vi "Help communication.vi"() -> ()   [LabVIEW 2018]
panel:
  out "EN help":string="The Channel selector is used to choose the type of communication between S4ICS and its clients.\nThe \"Inner TCP/IP\" option is implemented within the S4ICS program while the others are in the \"S4ICS InterComm.vi\" VI, opened and closed by S4ICS transparently for the user, unless the Local Panel option is selected. Local Panel is a GUI that allows local interactivity with SPARC4, replacing remote clients.\nThe Address, Port and Timeout configuration parameters are shared with TCP/IP, MQTT and ZeroMQ protocols.\nMQTT\nMQTT clients must connect to the broker indicated in Address and publish to topic \"lna/instrument/sparc4/command\" to send commands and subscribe to topic \"lna/instrument/sparc4/status\" to receive status message from S4ICS.\nZeroMQ\nZeroMQ customers..." caption="COMMUNICATION SELECTOR"
  out "PT help":string="O seletor Channel é usado para escolher o tipo de comunicação entre o S4ICS e seus clientes.\nA opção \"Inner TCP/IP\" está implementada dentro do programa S4ICS enquanto as demais no VI \"S4ICS InterComm.vi\", aberto e fechado pelo S4ICS de forma transparente para o usuário, exceto se a opção Local Panel for selecionada. Local Panel é uma GUI que permite interatividade local com o SPARC4, substituindo clientes remotos.\nOs parâmetros de configuração Address, Port e Timeout são compartilhados com os protocolos TCP/IP, MQTT e ZeroMQ.\nMQTT\nOs clientes MQTT devem se conectar ao broker indicado em Address e publicar no tópico \"lna/instrument/sparc4/command\" para enviar comandos e assinar o tópico \"lna/instrument/sparc4/status\" para receber a mensagem de status do S4ICS.\nZeroMQ\nOs clientes ZeroMQ..." caption="SELETOR DE COMUNICAÇAO"
  in  "ok":bool
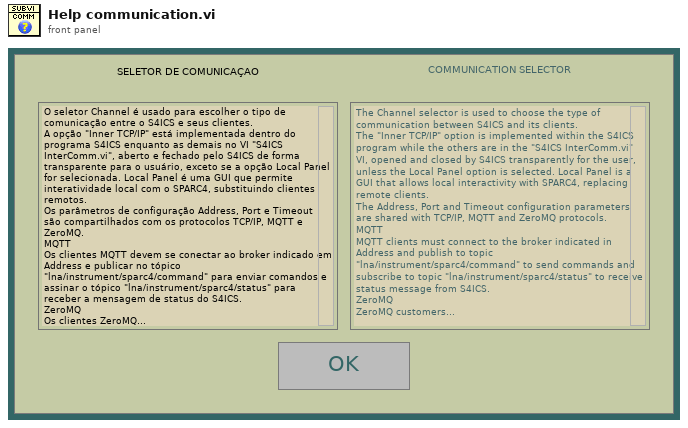
[diagram p1: front panel]
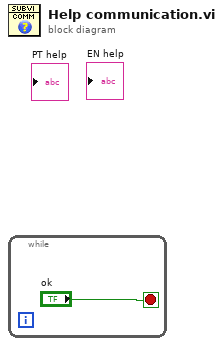
[diagram p0: block diagram]
diagram:
  n1 = while {
    stop <- "ok" stop-if-true
  }
